vi "Execute State.vi"(8 "error in (no error)":errorcluster, 9 "Data":variant, 10 "State":string, 11 "ExampleSimpleRootModel in":refnum<class "SimpleRootModel.lvclass">) -> (0 "error out":errorcluster, 3 "ExampleSimpleRootModel out":refnum<class "SimpleRootModel.lvclass">)   [LabVIEW 2017, in "MVAExamples.lvlib" / "SimpleRootModel.lvclass"]
uses:
  SimpleRootModel.lvclass
  C:/Git/mva-framework/Source/Framework/IModel/IModel/IModel.lvclass
  SimpleRootModel.lvclass/SimpleRootModel.ctl
  <vilib>/ActorFramework/Actor/Actor.lvclass/Actor.ctl
  <vilib>/ActorFramework/Message Enqueuer/Message Enqueuer.lvclass/Message Enqueuer.ctl
  Source/Framework/IModel/IModel/IModel.lvclass/IModel.ctl
  Source/Framework/IMediator/PublishRequest/PublishRequest.lvclass/PublishRequest.ctl
  Source/Framework/AbstractMessages/PreAddressedMsg/PreAddressedMsg.lvclass/PreAddressedMsg.ctl
  Source/Framework/IMediator/IMediator Messages/Publish Msg/Publish Msg.lvclass/Publish Msg.ctl
  Source/Framework/IMediator/IMediator Messages/Publish Msg/Send Pre-Addressed Publish.vi
  Source/Framework/IObserver/IObserver/Read Unique ID.vi
  Source/Framework/IMediator/PublishRequest/Pack Publish Request.vi
  <vilib>/ActorFramework/Message Enqueuer/Enqueue.vi
  Source/Framework/AbstractMessages/PreAddressedMsg/Read Return Address.vi
  <vilib>/ActorFramework/Actor/Read Self Enqueuer.vi
  <vilib>/ActorFramework/Message Enqueuer/Init from Existing Queue.vi
  Source/Framework/IModel/IModel/IModel.lvclass
  C:/Git/mva-framework/Source/Framework/IObserver/IObserver/IObserver.lvclass
  Source/Framework/IObserver/IObserver/IObserver.lvclass
  C:/Program Files (x86)/National Instruments/LabVIEW 2017/vi.lib/ActorFramework/Actor/Actor.lvclass
  Source/Framework/IMediator/IMediator Messages/Publish Msg/Publish Msg.lvclass
  C:/Git/mva-framework/Source/Framework/AbstractMessages/PreAddressedMsg/PreAddressedMsg.lvclass
  C:/Program Files (x86)/National Instruments/LabVIEW 2017/vi.lib/ActorFramework/Message/Message.lvclass
  <vilib>/ActorFramework/Message Priority Queue/Priority Enqueue.vi
  <vilib>/ActorFramework/Message Enqueuer/Message Enqueuer.lvclass
  Source/Framework/IMediator/PublishRequest/PublishRequest.lvclass
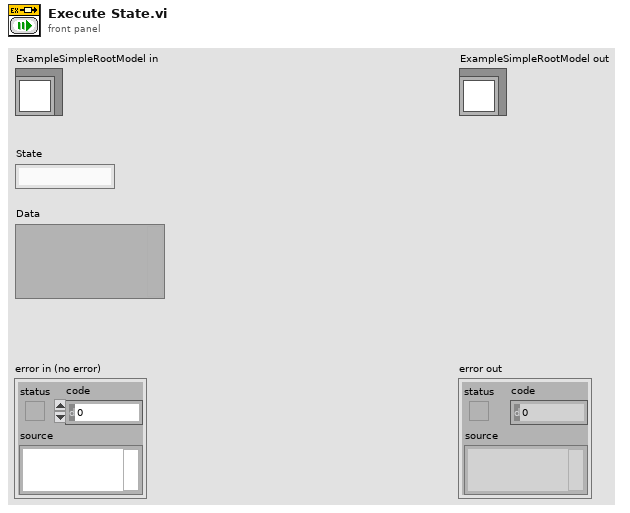
[diagram p1: front panel]
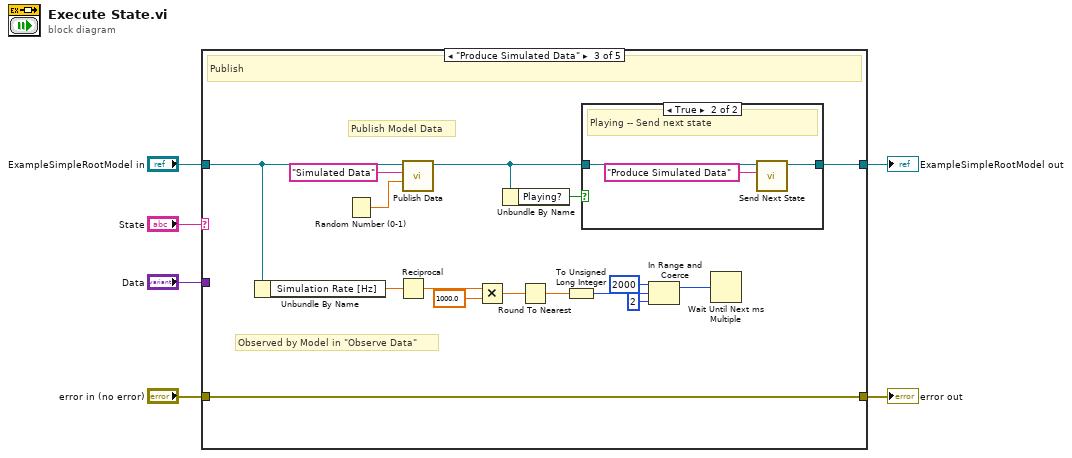
[diagram p0: block diagram]
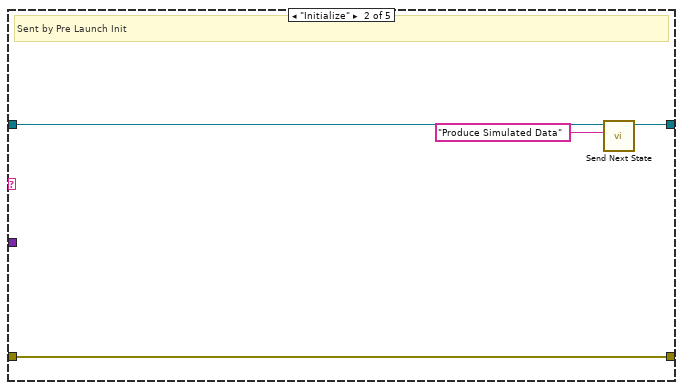
[diagram p3: hidden frame]
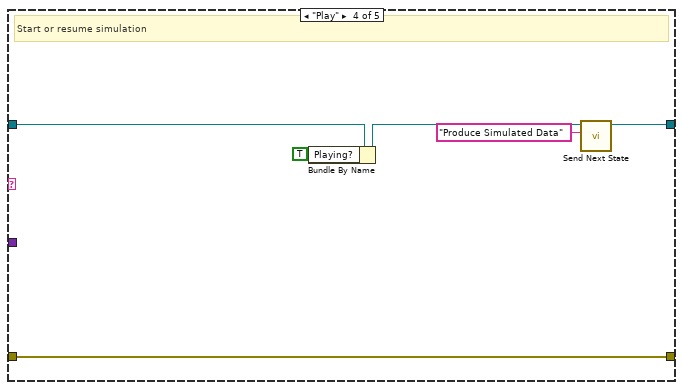
[diagram p5: hidden frame]
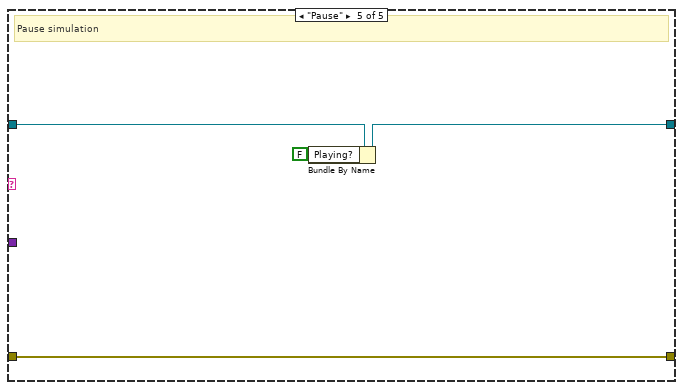
[diagram p6: hidden frame]
diagram:
  n1 = case shown="\"Produce Simulated Data\"" "State" {
    tunnel: [w7 w12 w28 w35 w39] -> w5
    tunnel: [w8 w10 w27 w34 w41] -> w3
    tunnel: "ExampleSimpleRootModel in" -> [w8 w11 w24 w38 w42]
    tunnel: "error in (no error)" -> [w7 w12 w28 w35 w39]
    tunnel: "Data" -> [_ _ _ _ _]
    frame Default {
      # "Unknown State Request"
    }
    frame "Initialize" {
      # "Sent by Pre Launch Init"
      n2 = call "Send Next State.vi"("State"="Produce Simulated Data", "ExampleSimpleRootModel in"=w11) -> ("ExampleSimpleRootModel out"=w10:refnum<class "SimpleRootModel.lvclass">)  [unwired: 8 in, 1 out]
    }
    frame "Produce Simulated Data" {
      # "Publish Model Data"
      # "Observed by Model in \"Observe Data\""
      # "Publish"
      n3 = Unbundle By Name(w24) -> ("Simulation Rate [Hz]"=w23:dbl)
      n4 = Random Number (0-1)() -> (number: 0 to 1=w25:dbl)
      n5 = Reciprocal(x=w23) -> (1/x=w22:dbl)
      n6 = call "Publish Data.vi"("Data to Publish"=w25, "Datum Name"="Simulated Data", "IModel in"=w24) -> ("IModel out"=w14:refnum<class "SimpleRootModel.lvclass">)  [unwired: 7 in, 1 out]
      n7 = Multiply(x=w22, y=1000.0) -> (x*y=w20:dbl)
      n8 = Unbundle By Name(w14) -> ("Playing?"=w13:bool)
      n9 = Round To Nearest(number=w20) -> (nearest integer value=w18:dbl)
      n10 = To Unsigned Long Integer(number=w18) -> (unsigned 32bit integer=w19:u32)
      n11 = case shown="True" w13 {
        tunnel: [w29 w32] -> w27
        tunnel: w14 -> [w29 w30]
        frame False {
          # "Paused -- Stop sending message to self"
        }
        frame True {
          # "Playing -- Send next state"
          n12 = call "Send Next State.vi"("State"="Produce Simulated Data", "ExampleSimpleRootModel in"=w30) -> ("ExampleSimpleRootModel out"=w32:refnum<class "SimpleRootModel.lvclass">)  [unwired: 8 in, 1 out]
        }
      }
      n13 = In Range and Coerce(upper limit=u32 2000, x=w19, lower limit=u32 2) -> (coerced(x)=w17:u32)  [unwired: 1 out]
      n14 = Wait Until Next ms Multiple(millisecond multiple=w17) -> ()  [unwired: 1 out]
    }
    frame "Play" {
      # "Start or resume simulation"
      n15 = Bundle By Name(cluster=w38, "Playing?"=TRUE ("Play?")) -> (w37:refnum<class "SimpleRootModel.lvclass">)
      n16 = call "Send Next State.vi"("State"="Produce Simulated Data", "ExampleSimpleRootModel in"=w37) -> ("ExampleSimpleRootModel out"=w34:refnum<class "SimpleRootModel.lvclass">)  [unwired: 8 in, 1 out]
    }
    frame "Pause" {
      # "Pause simulation"
      n17 = Bundle By Name(cluster=w42, "Playing?"=FALSE ("Play?")) -> (w41:refnum<class "SimpleRootModel.lvclass">)
    }
  }
  "error out" <- w5
  "ExampleSimpleRootModel out" <- w3
